vi "Send.vi"(8 "error in (no error)":errorcluster, 10 "Message":string, 11 "Fake ILC in":refnum<class "Fake ILC.lvclass">) -> (0 "error out":errorcluster, 3 "Fake ILC out":refnum<class "Fake ILC.lvclass">)   [LabVIEW 2015, in "Fake ILC.lvclass"]
uses:
  Fake ILC.lvclass
  Fake ILC.lvclass/Fake ILC.ctl
  <userlib>/Common/ILC/ILC/ILC.lvclass/ILC.ctl
  <userlib>/Common/ILC/ILC/ILC.lvclass
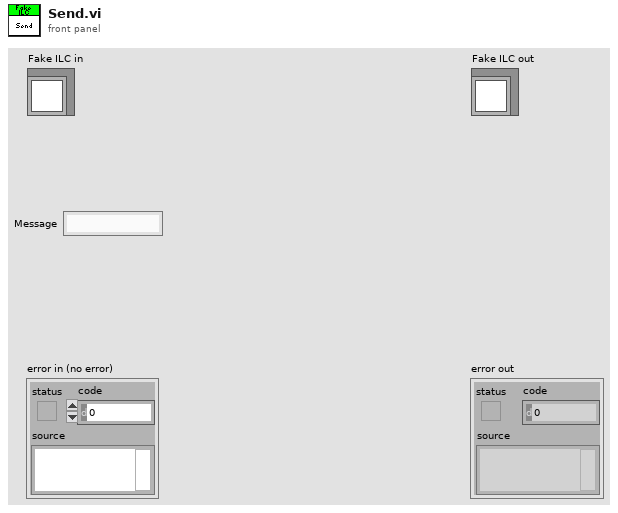
[diagram p1: front panel]
types:
  T1 = typedef "ILCCommon.lvlib/ILCTypedefs.lvlib/ADC Settings.ctl" = cluster{"Input Channels":T2, "Scan Rate (Hz) ":T3, "PGA Gain Coefficient":u8}
  T2 = typedef "ILCCommon.lvlib/ILCConfiguration.lvlib/Input Channels.ctl" = enum16{"Channel 0", "3 Channels", "5 Channels"}
  T3 = typedef "ILCCommon.lvlib/ILCConfiguration.lvlib/Scan Rates.ctl" = enum16{"50", "60", "100", "120", "200", "240", "300", "400", "480", "600", "1200", "2400", "4800"}
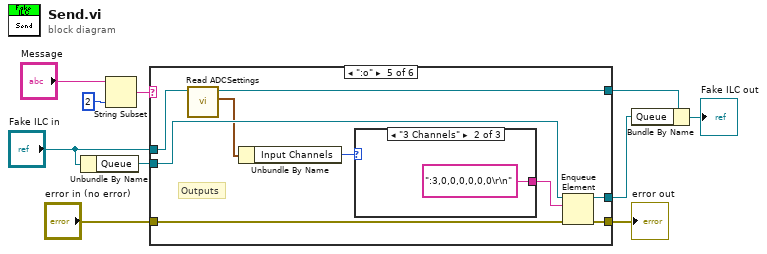
[diagram p0: block diagram]
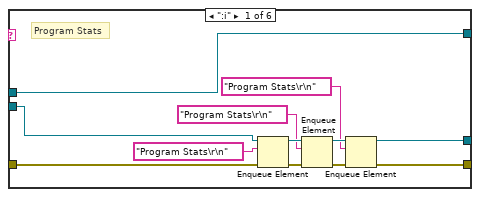
[diagram p2: hidden frame]
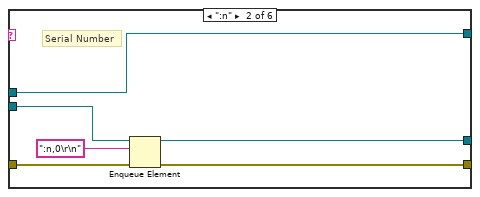
[diagram p3: hidden frame]
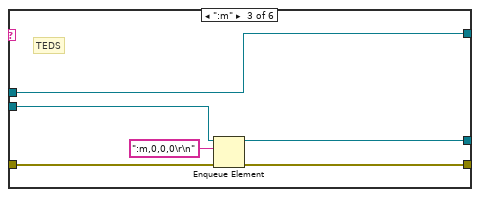
[diagram p4: hidden frame]
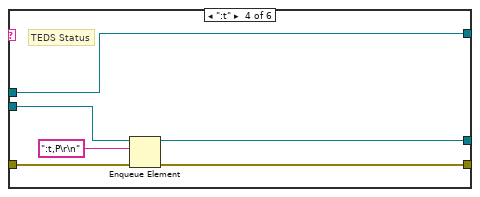
[diagram p5: hidden frame]
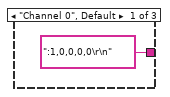
[diagram p6: hidden frame]
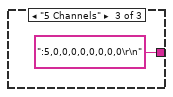
[diagram p7: hidden frame]
diagram:
  n1 = Unbundle By Name("Fake ILC in") -> ("Queue"=w5:refnum<queue>)
  n2 = String Subset(string="Message", length (rest)=2 ("length (rest)")) -> (substring=w7:string)  [unwired: 1 in]
  n3 = case shown="\":o\"" w7 {
    tunnel: [w20 w26 w33 w39 w48 w53] -> w3
    tunnel: "error in (no error)" -> [w19 w27 w34 w40 w49 w53]
    tunnel: w5 -> [w18 w28 w31 w37 w46 w54]
    tunnel: [w15 w25 w32 w38 w47 w54] -> w4
    tunnel: "Fake ILC in" -> [w11 w23 w29 w35 w45 w55]
    tunnel: [w11 w23 w29 w35 w44 w55] -> w1
    frame ":i" {
      # "Program Stats"
      n4 = Enqueue Element(queue=w18, element="Program Stats\r\n", error in (no error)=w19) -> (queue out=w17:refnum<queue>, error out=w22:errorcluster)  [unwired: 1 in, 1 out]
      n5 = Enqueue Element(queue=w17, element="Program Stats\r\n", error in (no error)=w22) -> (queue out=w16:refnum<queue>, error out=w21:errorcluster)  [unwired: 1 in, 1 out]
      n6 = Enqueue Element(queue=w16, element="Program Stats\r\n", error in (no error)=w21) -> (queue out=w15:refnum<queue>, error out=w20:errorcluster)  [unwired: 1 in, 1 out]
    }
    frame ":n" {
      # "Serial Number"
      n7 = Enqueue Element(queue=w28, element=":n,0\r\n", error in (no error)=w27) -> (queue out=w25:refnum<queue>, error out=w26:errorcluster)  [unwired: 1 in, 1 out]
    }
    frame ":m" {
      # "TEDS"
      n8 = Enqueue Element(queue=w31, element=":m,0,0,0\r\n", error in (no error)=w34) -> (queue out=w32:refnum<queue>, error out=w33:errorcluster)  [unwired: 1 in, 1 out]
    }
    frame ":t" {
      # "TEDS Status"
      n9 = Enqueue Element(queue=w37, element=":t,P\r\n", error in (no error)=w40) -> (queue out=w38:refnum<queue>, error out=w39:errorcluster)  [unwired: 1 in, 1 out]
    }
    frame ":o" {
      # "Outputs"
      n10 = call <userlib>:"Read ADCSettings.vi"("ILC in"=w45) -> ("ADC Settings"=w43:T1, "ILC out"=w44:refnum<class "Fake ILC.lvclass">)  [unwired: 9 in]
      n11 = Unbundle By Name(w43) -> ("Input Channels"=w42:T2)
      n12 = case shown="\"3 Channels\"" w42 {
        tunnel: [":1,0,0,0,0\r\n" ("element") ":3,0,0,0,0,0,0\r\n" ("element") ":5,0,0,0,0,0,0,0,0\r\n" ("element")] -> w41
        frame "Channel 0", Default {
        }
        frame "3 Channels" {
        }
        frame "5 Channels" {
        }
      }
      n13 = Enqueue Element(queue=w46, element=w41, error in (no error)=w49) -> (queue out=w47:refnum<queue>, error out=w48:errorcluster)  [unwired: 1 in, 1 out]
    }
    frame Default {
    }
  }
  "error out" <- w3
  n14 = Bundle By Name(cluster=w1, "Queue"=w4) -> (→"Fake ILC out":refnum<class "Fake ILC.lvclass">)
